vi "DecodeError.vi"(2 "Error Code (0)":i32, 3 "resource name":string="USB0::0x1313::0x8078::P0005368::INSTR") -> (0 "error out":errorcluster {"code" format="%.0x"}, 1 "Error Message":string)   [LabVIEW 2015]
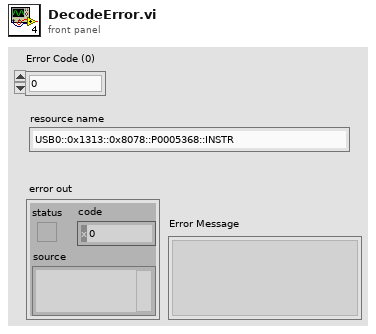
[diagram p1: front panel]
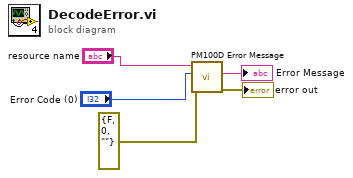
[diagram p0: block diagram]
diagram:
  n1 = call "PM100D Error Message.vi"("error in (no error)"=errorcluster {"status"=FALSE, "code"=0, "source"=""}, "Error Code (0)"="Error Code (0)", "instrument handle"="resource name") -> ("error out"=→"error out":errorcluster, "Error Message"=→"Error Message":string)  [unwired: 6 in, 1 out]
